vi "Result View.vi"(11 "Result Model":refnum<class "Result Model.lvclass">) -> ()   [LabVIEW 2020, in "Test Result View.lvclass"]
uses:
  Test Result View.lvclass
  User Interface/Result Model/Tree Item Filter.ctl
  User Interface/Result Model/Result Model.lvclass
panel:
  in  "Test Results":string[](tree)
  in  "Filter fails":bool
  out "Description":string
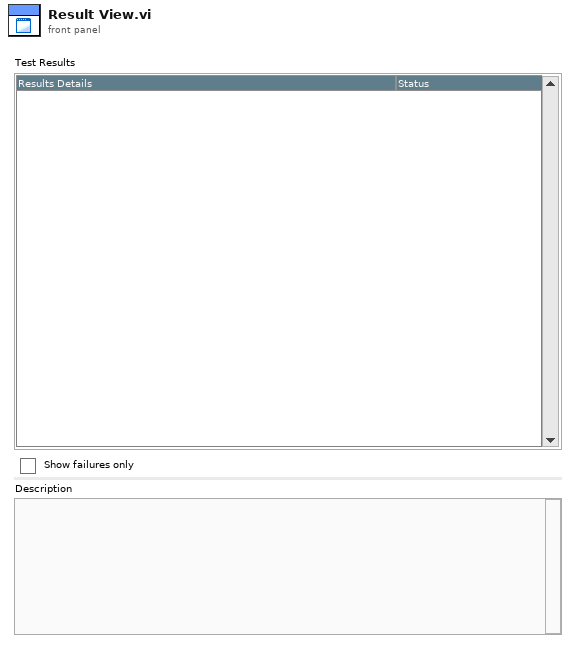
[diagram p1: front panel]
types:
  T1 = typedef "Result Model.lvclass/Tree Item Filter.ctl" = enum16{"All", "Only Fails", "Fails or else Not Executed"}
  T2 = enum32{"Invalid", "Standard", "Closed", "Hidden", "Minimized", "Maximized"}
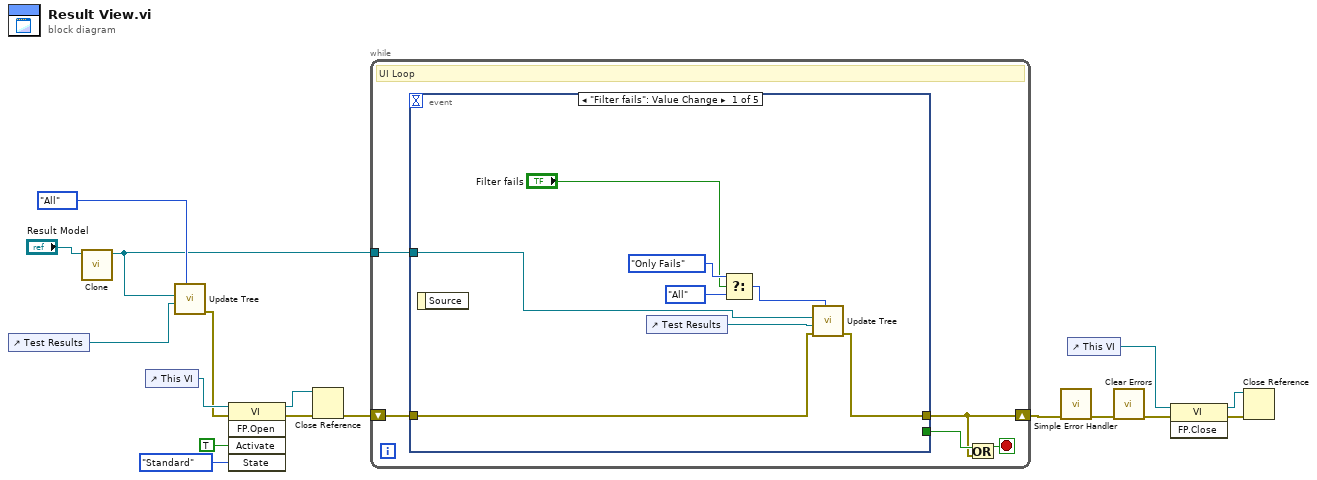
[diagram p0: block diagram]
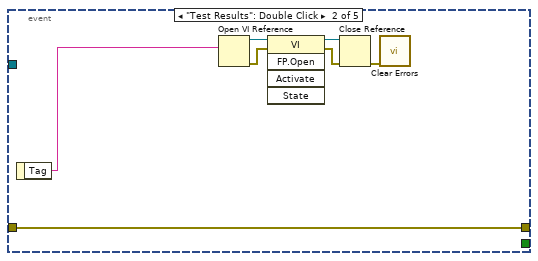
[diagram p2: hidden frame]
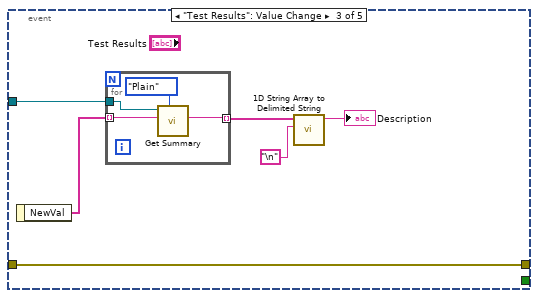
[diagram p3: hidden frame]
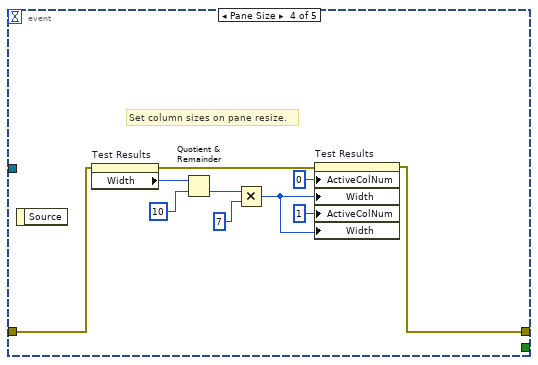
[diagram p4: hidden frame]
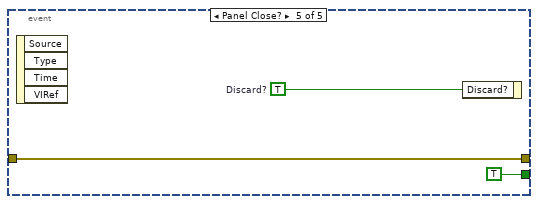
[diagram p5: hidden frame]
diagram:
  n1 = control-ref of="Test Results"() -> (w5:refnum<vi>)
  n2 = call "Clone.vi"("Result Model by Reference in"="Result Model") -> ("Result Model by Reference out"=w1:refnum<class "Result Model.lvclass">)  [unwired: 9 in, 1 out]
  n3 = control-ref of="This VI"() -> (w9:refnum<vi>)
  n4 = call "Update Tree.vi"("Filter"=Tree_Item_Filter."All", "Test Tree"=w5, "Result Model"=w1) -> ("error out"=w4:errorcluster)  [unwired: 8 in]
  n5 = invoke on="Invoke Node" class="VI" method="FP.Open"(reference=w9, error in=w4, "Activate"=TRUE ("Activate?"), "State"=T2."Standard") -> (reference out=w11:refnum<vi>, error out=w10:errorcluster)  [unwired: 1 in, 3 out]
  n6 = Close Reference(reference=w11, error in (no error)=w10) -> (error out=w6:errorcluster)
  n7 = while {
    shift-right: [w19] -> w17
    shift-left: w6 -> [w22]
    tunnel: w1 -> [w18]
    stop <- w20 stop-if-true
    # "UI Loop"
    n8 = event shown="[0] \"Filter fails\": Value Change" {
      selector: _ -> [_ _ _ _ _]
      dyn-events: _ -> [_ _ _ _ _]
      timeout: _ -> [_ _ _ _ _]
      tunnel: w22 -> [w24 w37 w43 w48 w59]
      tunnel: [w25 w37 w43 w49 w59] -> w19
      tunnel: [_ _ _ _ TRUE] -> w21
      tunnel: w18 -> [w23 _ w39 _ _]
      event "Filter fails": Value Change {
        n9 = event-data() -> ()  [unwired: 1 in, 1 out]
        n10 = control-ref of="Test Results"() -> (w29:refnum<vi>)
        n11 = Select(t=Tree_Item_Filter."Only Fails" ("Filter"), s="Filter fails", f=Tree_Item_Filter."All" ("Filter")) -> (s? t:f=w30:T1)
        n12 = call "Update Tree.vi"("Filter"=w30, "error in (no error)"=w24, "Test Tree"=w29, "Result Model"=w23) -> ("error out"=w25:errorcluster)  [unwired: 7 in]
      }
      event "Test Results": Double Click {
        n13 = event-data() -> ("Tag"=w31:string)  [unwired: 1 in]
        n14 = Open VI Reference(vi path=w31) -> (vi reference=w32:refnum<vi>, error out=w33:errorcluster)  [unwired: 5 in]
        n15 = invoke class="VI" method="FP.Open"(reference=w32, error in=w33) -> (reference out=w35:refnum<vi>, error out=w34:errorcluster)  [unwired: 3 in, 3 out]
        n16 = Close Reference(reference=w35, error in (no error)=w34) -> (error out=w36:errorcluster)
        n17 = call <vilib>:"Clear Errors.vi"("error in (no error)"=w36) -> ()  [unwired: 5 in, 2 out]
      }
      event "Test Results": Value Change {
        n18 = event-data() -> ("NewVal"=w40:string[])  [unwired: 1 in]
        n19 = for {
          tunnel: w39 -> [w47]
          tunnel: w40 -> [w46] mode=indexing
          tunnel: [w45] -> w42 mode=indexing
          n20 = call "Get Summary.vi"("Style"=enum16{"Diff", "Plain"}."Plain", "Item"=w46, "Result Model by Reference In"=w47) -> ("Summary"=w45:string)  [unwired: 7 in, 1 out]
        }
        n21 = call <vilib>:"1D String Array to Delimited String.vi"("delimiter"="\n", "string array"=w42) -> ("delimited string"=→"Description":string)  [unwired: 9 in]
      }
      event Pane Size {
        # "Set column sizes on pane resize."
        n22 = event-data() -> ()  [unwired: 1 in, 1 out]
        n23 = property on="Test Results" class="Tree (strict)"(error in=w48) -> (error out=w50:errorcluster, "Width"=w51:u32)  [unwired: 1 in, 1 out]
        n24 = Quotient & Remainder(x=w51, y=u32 10) -> (floor(x/y)=w55:u32)  [unwired: 1 out]
        n25 = Multiply(x=w55, y=u32 7) -> (x*y=w52:u32)
        n26 = property on="Test Results" class="Tree (strict)"(error in=w50, "ActiveColNum"=0 ("Active Cell:Active Column Number"), "Width"=w52, "ActiveColNum"=1 ("Active Cell:Active Column Number"), "Width"=w52) -> (error out=w49:errorcluster)  [unwired: 1 in, 1 out]
      }
      event Panel Close? {
        w60 = TRUE  # Discard?
        n27 = event-data() -> ()  [unwired: 1 in, 4 out]
        n28 = event-data ("Event Filter Node")("Discard?"=w60) -> ()  [unwired: 1 in, 1 out]
      }
    }
    n29 = Or(x=w21, y=w19) -> (x .or. y?=w20:bool)
  }
  n30 = call <vilib>:"Simple Error Handler.vi"("error in (no error)"=w17) -> ("error out"=w13:errorcluster)  [unwired: 4 in, 4 out]
  n31 = control-ref of="This VI"() -> (w14:refnum<vi>)
  n32 = call <vilib>:"Clear Errors.vi"("error in (no error)"=w13) -> ("error out"=w12:errorcluster)  [unwired: 5 in, 1 out]
  n33 = invoke on="Invoke Node" class="VI" method="FP.Close"(reference=w14, error in=w12) -> (reference out=w16:refnum<vi>, error out=w15:errorcluster)  [unwired: 1 in, 1 out]
  n34 = Close Reference(reference=w16, error in (no error)=w15) -> ()  [unwired: 1 out]
